vi "ErrorHandlerMainLoop.vi"(0 "object in":refnum<class "Application.lvclass">, 5 "error in (no error)":errorcluster) -> (14 "object out":refnum<class "Application.lvclass">, 19 "error out":errorcluster)   [LabVIEW 2019, in "Application.lvclass"]
uses:
  Application.lvclass
panel:
  in  "Ignore Errors (Runtime)":i32[](array[numeric])
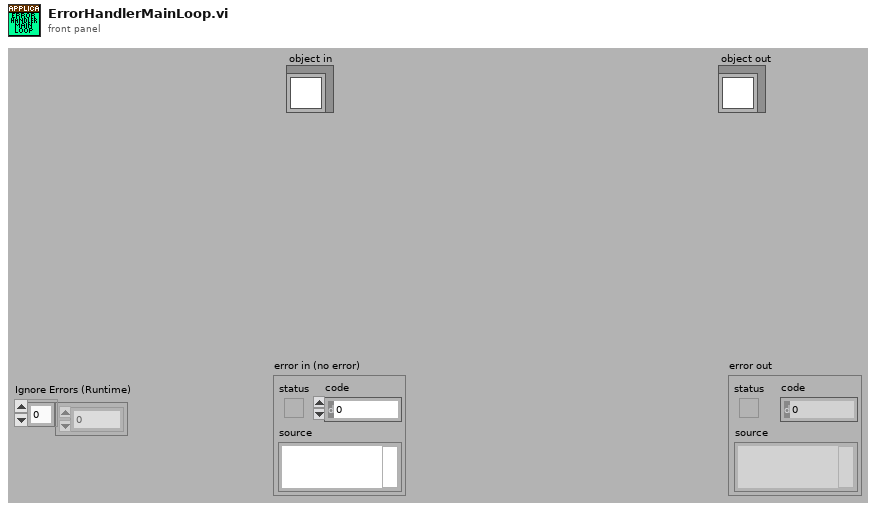
[diagram p1: front panel]
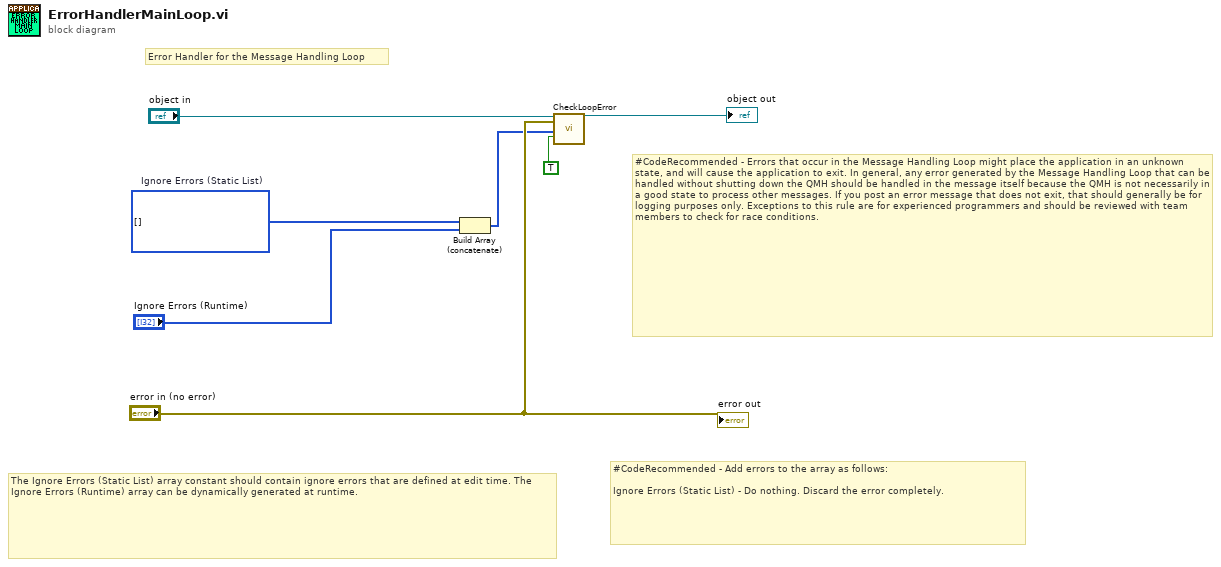
[diagram p0: block diagram]
diagram:
  w6 = i32[] []  # Ignore Errors (Static List)
  # "#CodeRecommended - Errors that occur in the Message Handling Loop might place the application in an unknown state, and will cause the application to exit. In general, any error generated by the Message Handling Loop that can be handled without shutting down the QMH should be handled in the message itself because the QMH is not necessarily in a good state to process other messages. If you post an error message that does not exit, that should generally be for logging purposes only. Exceptions to this rule are for experienced programmers and should be reviewed with team members to check for race conditions."
  # "The Ignore Errors (Static List) array constant should contain ignore errors that are defined at edit time. The Ignore Errors (Runtime) array can be dynamically generated at runtime."
  # "#CodeRecommended - Add errors to the array as follows:\n\nIgnore Errors (Static List) - Do nothing. Discard the error completely."
  # "Error Handler for the Message Handling Loop"
  n1 = Build Array (concatenate)(w6, "Ignore Errors (Runtime)") -> (w3:i32[])
  n2 = call-dynamic "CheckLoopError.vi"("object in"="object in", "error to process"="error in (no error)", "Ignore Errors"=w3, "Exit on Error? (F)"=TRUE) -> ("object out"=→"object out":refnum<class "Application.lvclass">)  [unwired: 14 in, 1 out]
  "error out" <- "error in (no error)"
